vi "MB demo test_v2.vi"() -> ()   [LabVIEW 2018, in "MB Relay.lvlib"]
uses:
  MB Relay.lvlib
  type defs/FGV enum.ctl
  <vilib>/ErrorRing/Error Ring.xnode
  <vilib>/NI/Modbus Library/API/Master/Modbus Master.lvclass
panel:
  out "index of element":i32
  in  "Boolean":bool
  in  "5V enable":bool
  out "output array":bool[][](array[boolean])
  in  "All ON":bool
  in  "mux2-1(DMM I) encode":enum16{"DMM I (0.5)", "DMM I (12)"}(ring)
  in  "DMM I 0.5":bool
  out "short circuits":bool[](array[boolean])
  in  "mux6_1(3wires)_encode":T1(ring)
  in  "mux6-1(3 wires)":bool
  in  "SpareRelays":bool[](array[boolean])=[FALSE, FALSE, FALSE, FALSE, FALSE, FALSE, FALSE, FALSE, FALSE, FALSE, FALSE, FALSE, FALSE, FALSE, FALSE]
  in  "SpareRelay":bool
  in  "MB relay01":bool[](array[boolean])=[FALSE, FALSE, FALSE, FALSE, FALSE, FALSE, FALSE, FALSE, FALSE, FALSE, FALSE, FALSE, FALSE, FALSE, FALSE, FALSE]
  in  "MB relay01":bool
  in  "mux10_1(x6)_encode":T2(ring)
  in  "demux1_10(x6)_encode":T3(ring)
  in  "Read Optos":bool
  out "counter":u16
  in  "ALL OFF":bool
  in  "mux10-1":bool
  in  "demux1-10":bool
  in  "unit ID":u8=50
  in  "stop":bool
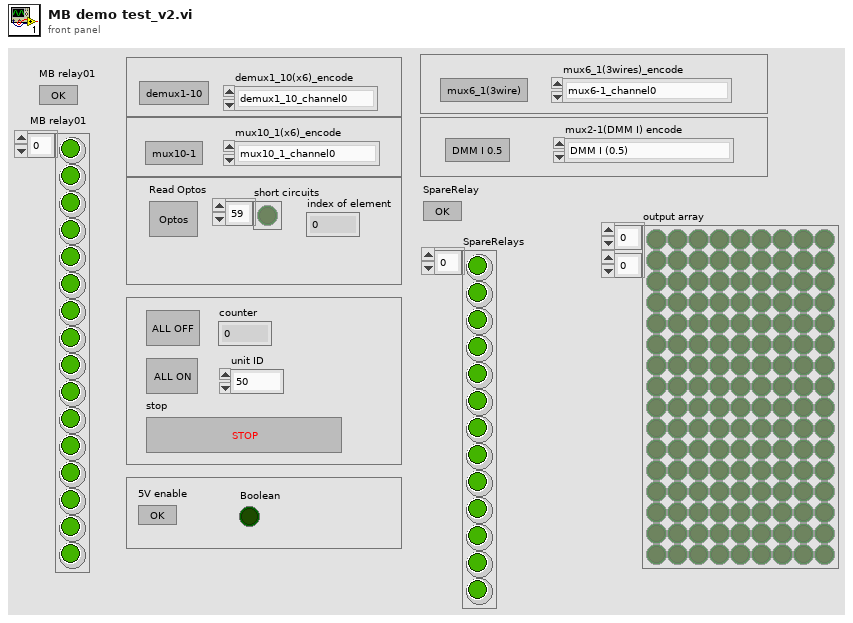
[diagram p1: front panel]
types:
  T1 = enum16{"mux6-1_channel0", "mux6_1_channel1_0", "mux6_1_channel1_1", "mux6-1_channel1_2", "mux6_1_channel1_3", "mux6_1_channel2_0", "mux6_1_channel2_1", "mux6_1_channel2_2", "mux6_1_channel2_3", "mux6_1_channel3_0", "mux6_1_channel3_1", "mux6_1_channel3_2", "mux6_1_channel3_3", "mux6_1_channel4_0", "mux6_1_channel4_1", "mux6_1_channel4_2", "mux6_1_channel4_3", "mux6_1_channel5_0", "mux6_1_channel5_1", "mux6_1_channel5_2", "mux6_1_channel5_3", "mux6_1_channel6_0", "mux6_1_channel6_1", "mux6_1_channel6_2", "mux6_1_channel6_3"}
  T2 = enum16{"mux10_1_channel0", "mux10_1_channel1", "mux10_1_channel2", "mux10_1_channel3", "mux10_1_channel4", "mux10_1_channel5", "mux10_1_channel6", "mux10_1_channel7", "mux10_1_channel8", "mux10_1_channel9", "mux10_1_channel10"}
  T3 = enum16{"demux1_10_channel0", "demux1_10_channel1", "demux1_10_channel2", "demux1_10_channel3", "demux1_10_channel4", "demux1_10_channel5", "demux1_10_channel6", "demux1_10_channel7", "demux1_10_channel8", "demux1_10_channel9", "demux1_10_channel10"}
  T4 = typedef "MB Relay.lvlib/FGV enum.ctl" = enum16{"Write", "Read", "All OFF", "All ON"}
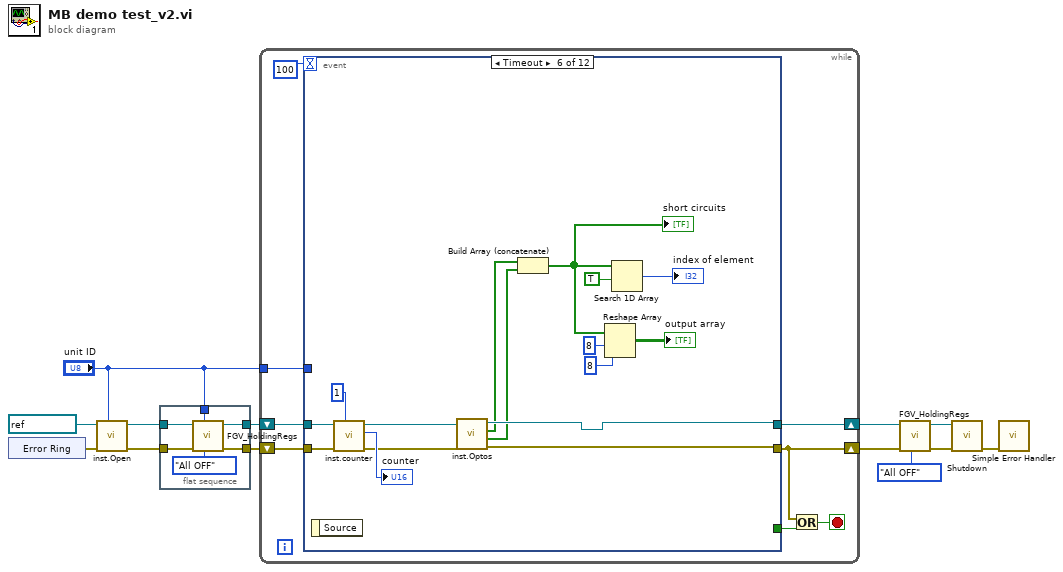
[diagram p0: block diagram]
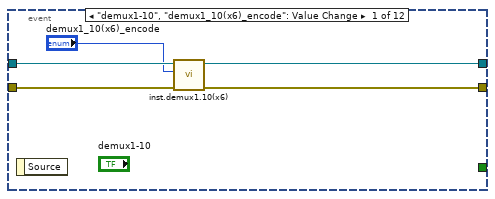
[diagram p2: hidden frame]
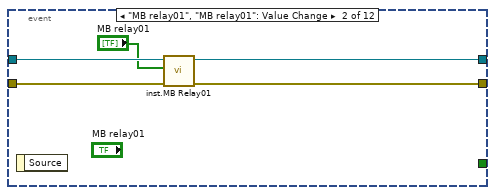
[diagram p3: hidden frame]
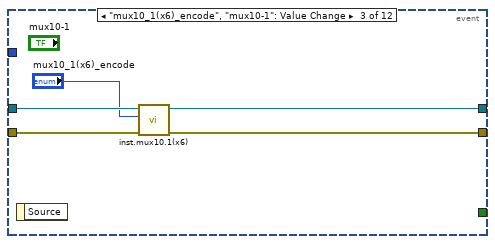
[diagram p4: hidden frame]
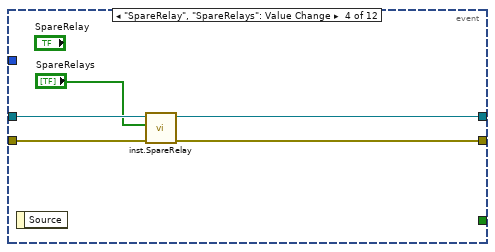
[diagram p5: hidden frame]
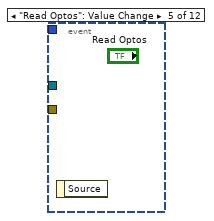
[diagram p6: hidden frame]
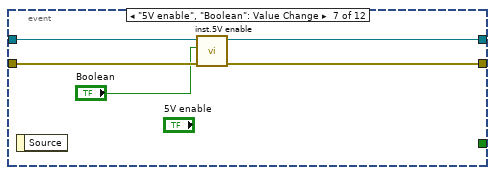
[diagram p7: hidden frame]
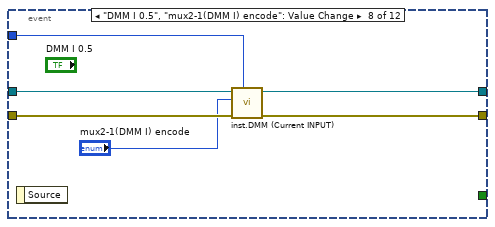
[diagram p8: hidden frame]
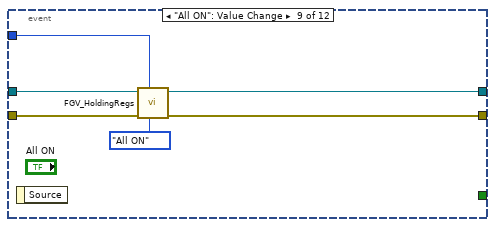
[diagram p9: hidden frame]
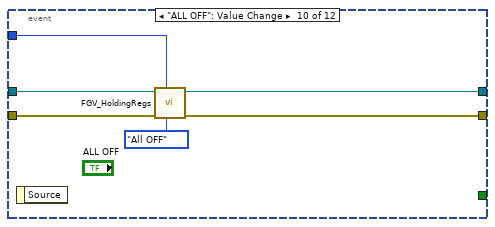
[diagram p10: hidden frame]
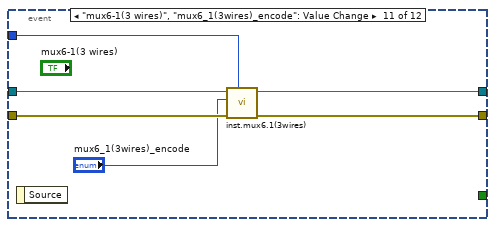
[diagram p11: hidden frame]
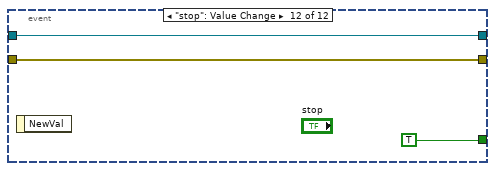
[diagram p12: hidden frame]
diagram:
  n1 = xnode "Error Ring"() -> ("error out"=w7:errorcluster)
  n2 = call "inst.Open.vi"("unit ID in"="unit ID", "error in (no error)"=w7, "VISA resource name"=refnum<visa-resource-name> "COM11") -> ("error out"=w11:errorcluster, "Modbus Master out"=w12:refnum<class "Modbus Master.lvclass">)  [unwired: 7 in]
  n3 = flat-sequence {
    tunnel: w12 -> [w19]
    tunnel: w11 -> [w18]
    tunnel: [w17] -> w10
    tunnel: [w16] -> w9
    tunnel: "unit ID" -> [w15]
    frame #0 {
      n4 = call "FGV_HoldingRegs.vi"("FGV_enum"=FGV_enum."All OFF", "unit ID"=w15, "error in (no error)"=w18, "Modbus master in"=w19) -> ("error out"=w16:errorcluster, "Modbus master out"=w17:refnum<class "Modbus Master.lvclass">)  [unwired: 5 in, 1 out]
    }
  }
  n5 = while {
    shift-right: [w21] -> w6
    shift-left: w10 -> [w27]
    tunnel: "unit ID" -> [w25]
    shift-right: [w20] -> w5
    shift-left: w9 -> [w26]
    stop <- w22 stop-if-true
    n6 = event shown="[5] Timeout" {
      selector: _ -> [_ _ _ _ _ _ _ _ _ _ _ _]
      dyn-events: _ -> [_ _ _ _ _ _ _ _ _ _ _ _]
      timeout: 100 -> [_ _ _ _ _ _ _ _ _ _ _ _]
      tunnel: w27 -> [w32 w37 w42 w47 _ w61 w66 w74 w80 w86 w92 w95]
      tunnel: [_ _ _ _ _ _ _ _ _ _ _ TRUE] -> w23
      tunnel: w26 -> [w31 w34 w40 w46 _ w60 w68 w71 w79 w85 w89 w94]
      tunnel: [w29 w35 w39 w44 _ w52 w67 w73 w76 w84 w90 w94] -> w20
      tunnel: [w30 w36 w41 w45 _ w51 w65 w72 w75 w83 w91 w95] -> w21
      tunnel: w25 -> [_ _ _ _ _ _ _ w70 w78 w81 w88 _]
      event "demux1-10", "demux1_10(x6)_encode": Value Change {
        n7 = event-data() -> ()  [unwired: 1 in, 1 out]
        n8 = call "inst.demux1.10(x6).vi"("error in (no error)"=w31, "demux1_10(x6)_encode"="demux1_10(x6)_encode", "Modbus Master in"=w32) -> ("error out"=w29:errorcluster, "Modbus Master out"=w30:refnum<class "Modbus Master.lvclass">)  [unwired: 7 in]
      }
      event "MB relay01", "MB relay01": Value Change {
        n9 = event-data() -> ()  [unwired: 1 in, 1 out]
        n10 = call "inst.MB Relay01.vi"("error in (no error)"=w34, "MB relay01"="MB relay01", "Modbus Master in"=w37) -> ("error out"=w35:errorcluster, "Modbus Master out"=w36:refnum<class "Modbus Master.lvclass">)  [unwired: 7 in]
      }
      event "mux10_1(x6)_encode", "mux10-1": Value Change {
        n11 = event-data() -> ()  [unwired: 1 in, 1 out]
        n12 = call "inst.mux10.1(x6).vi"("error in (no error)"=w40, "mux10_1(x6)_encode"="mux10_1(x6)_encode", "Modbus Master in"=w42) -> ("error out"=w39:errorcluster, "Modbus Master out"=w41:refnum<class "Modbus Master.lvclass">)  [unwired: 7 in]
      }
      event "SpareRelay", "SpareRelays": Value Change {
        n13 = event-data() -> ()  [unwired: 1 in, 1 out]
        n14 = call "inst.SpareRelay.vi"("error in (no error)"=w46, "SpareRelays"="SpareRelays", "Modbus Master in"=w47) -> ("error out"=w44:errorcluster, "Modbus Master out"=w45:refnum<class "Modbus Master.lvclass">)  [unwired: 7 in]
      }
      event "Read Optos": Value Change {
        n15 = event-data() -> ()  [unwired: 1 in, 1 out]
      }
      event Timeout {
        n16 = event-data() -> ()  [unwired: 1 in, 1 out]
        n17 = call "inst.counter.vi"("unit ID(1)"=u8 1, "error in (no error)"=w60, "Modbus master in"=w61) -> ("error out"=w53:errorcluster, "counter"=→"counter":u16, "Modbus master out"=w54:refnum<class "Modbus Master.lvclass">)  [unwired: 6 in]
        n18 = call "inst.Optos.vi"("error in (no error)"=w53, "Modbus master in"=w54) -> ("error out"=w52:errorcluster, "inputs"=w49:bool[], "short circuits"=w50:bool[], "Modbus master out"=w51:refnum<class "Modbus Master.lvclass">)  [unwired: 6 in]
        n19 = Build Array (concatenate)(w50, w49) -> (w48:bool[])
        "short circuits" <- w48
        n20 = Reshape Array(w48, 8 ("dimension size"), 8 ("dimension size")) -> (→"output array":bool[][])
        n21 = Search 1D Array(1D array=w48, element=TRUE) -> (index of element=→"index of element":i32)  [unwired: 1 in]
      }
      event "5V enable", "Boolean": Value Change {
        n22 = event-data() -> ()  [unwired: 1 in, 1 out]
        n23 = call "inst.5V enable.vi"("error in (no error)"=w68, "5V enable"="Boolean", "Modbus Master in"=w66) -> ("error out"=w67:errorcluster, "Modbus Master out"=w65:refnum<class "Modbus Master.lvclass">)  [unwired: 7 in]
      }
      event "DMM I 0.5", "mux2-1(DMM I) encode": Value Change {
        n24 = event-data() -> ()  [unwired: 1 in, 1 out]
        n25 = call "inst.DMM (Current INPUT).vi"("unit ID"=w70, "error in (no error)"=w71, "mux2-1(DMM I) encode"="mux2-1(DMM I) encode", "Modbus Master in"=w74) -> ("error out"=w73:errorcluster, "Modbus Master out"=w72:refnum<class "Modbus Master.lvclass">)  [unwired: 6 in]
      }
      event "All ON": Value Change {
        n26 = event-data() -> ()  [unwired: 1 in, 1 out]
        n27 = call "FGV_HoldingRegs.vi"("FGV_enum"=FGV_enum."All ON", "unit ID"=w78, "error in (no error)"=w79, "Modbus master in"=w80) -> ("error out"=w76:errorcluster, "Modbus master out"=w75:refnum<class "Modbus Master.lvclass">)  [unwired: 5 in, 1 out]
      }
      event "ALL OFF": Value Change {
        n28 = event-data() -> ()  [unwired: 1 in, 1 out]
        n29 = call "FGV_HoldingRegs.vi"("FGV_enum"=FGV_enum."All OFF", "unit ID"=w81, "error in (no error)"=w85, "Modbus master in"=w86) -> ("error out"=w84:errorcluster, "Modbus master out"=w83:refnum<class "Modbus Master.lvclass">)  [unwired: 5 in, 1 out]
      }
      event "mux6-1(3 wires)", "mux6_1(3wires)_encode": Value Change {
        n30 = event-data() -> ()  [unwired: 1 in, 1 out]
        n31 = call "inst.mux6.1(3wires).vi"("unit ID"=w88, "error in (no error)"=w89, "mux6_1(3wires)_encode"="mux6_1(3wires)_encode", "Modbus Master in"=w92) -> ("error out"=w90:errorcluster, "Modbus Master out"=w91:refnum<class "Modbus Master.lvclass">)  [unwired: 6 in]
      }
      event "stop": Value Change {
        n32 = event-data() -> ()  [unwired: 1 in, 1 out]
      }
    }
    n33 = Or(x=w20, y=w23) -> (x .or. y?=w22:bool)
  }
  n34 = call "FGV_HoldingRegs.vi"("FGV_enum"=FGV_enum."All OFF", "error in (no error)"=w5, "Modbus master in"=w6) -> ("error out"=w4:errorcluster, "Modbus master out"=w3:refnum<class "Modbus Master.lvclass">)  [unwired: 6 in, 1 out]
  n35 = call-dynamic "Shutdown.vi"("error in"=w4, "Modbus master in"=w3) -> ("error out"=w13:errorcluster)  [unwired: 9 in]
  n36 = call <vilib>:"Simple Error Handler.vi"("error in (no error)"=w13) -> ()  [unwired: 4 in, 5 out]
